vi "var_num_v1.vi"() -> ()   [LabVIEW 2009]
panel:
  out "Afisare valoare numerica":i16
  in  "Introducere valoare numerica":i32(knob) scale=0.0..100.0
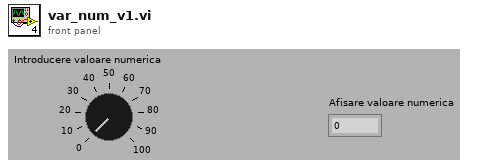
[diagram p1: front panel]
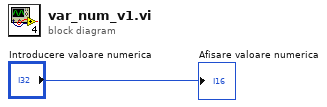
[diagram p0: block diagram]
diagram:
  "Afisare valoare numerica" <- "Introducere valoare numerica"
